vi "Logging Clear Tree.vi"(7 "TreeRef":refnum<vi>) -> (3 "TreeRef":refnum<vi>)   [LabVIEW 2012, in "femtoRoboLib.lvlib"]
doc: "Simply deletes all nodes from the provided Tree reference."
uses:
  femtoRoboLib.lvlib
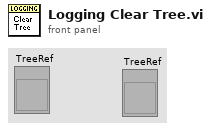
[diagram p1: front panel]
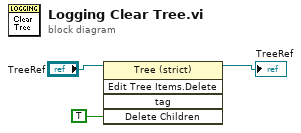
[diagram p0: block diagram]
diagram:
  n1 = invoke class="Tree (strict)" method="Edit Tree Items.Delete"(reference="TreeRef", "Delete Children"=TRUE ("Delete Children?")) -> (reference out=→"TreeRef":refnum<vi>)  [unwired: 3 in, 4 out]
